vi "Word cmd.vi"(6 "Word cmd":T3, 8 "Error In (no error)":errorcluster, 10 "Mathcad Output":T1, 11 "DesignRequest":T2) -> (0 "error out":errorcluster, 1 "Find-Replace":cluster{"Find":string, "Replace":string}[](array[cluster]))   [LabVIEW 2012, in "Design Server.lvlib"]
uses:
  Design Server.lvlib
  Word cmd.ctl
  Design Request.ctl
  Variable cluster.ctl
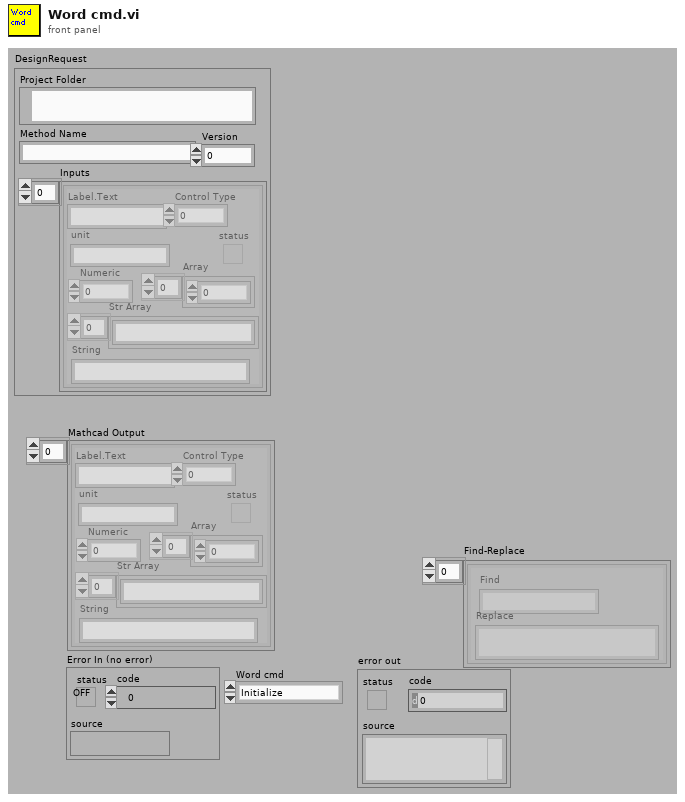
[diagram p1: front panel]
types:
  T1 = typedef "Design Server.lvlib/Variable cluster.ctl" = cluster{"Label.Text":string, "Control Type":u32, "Numeric":dbl, "Array":dbl[], "status":bool, "Str Array":string[], "String":string, "unit":string}[]
  T2 = typedef "Design Server.lvlib/Design Request.ctl" = cluster{"Project Folder":path, "Method Name":string, "Inputs":T1, "Version":i32}
  T3 = typedef "Design Server.lvlib/Word cmd.ctl" = enum16{"Initialize", "Create Reports", "Quit"}
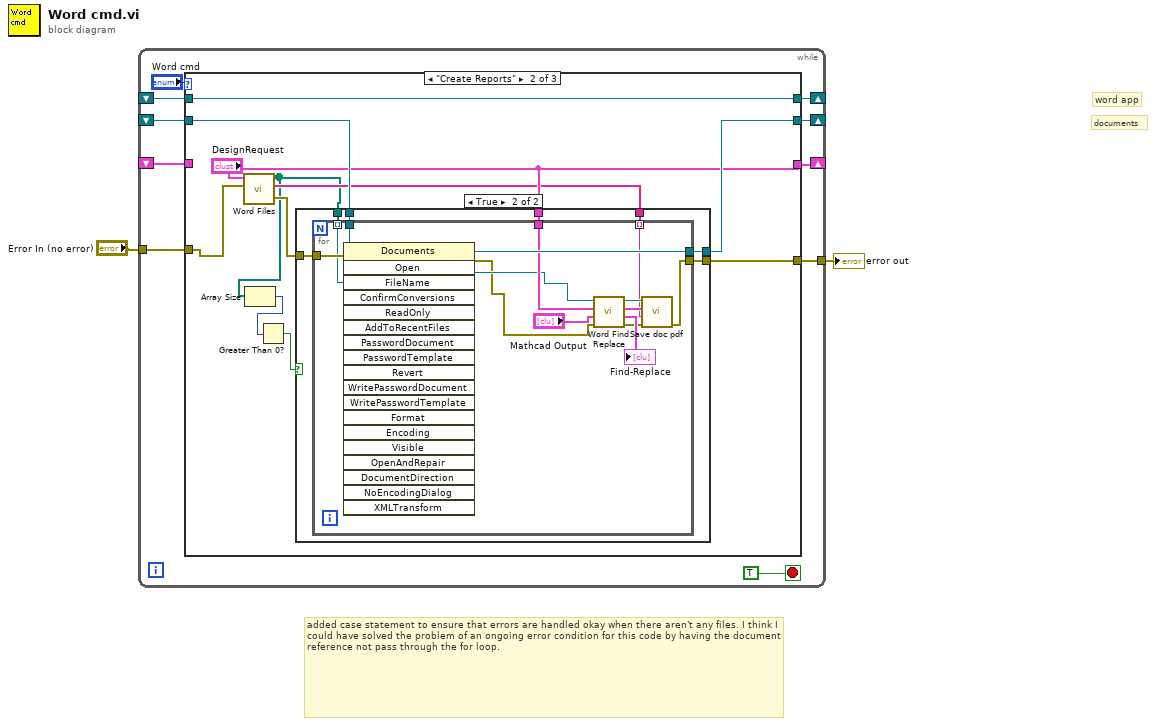
[diagram p0: block diagram]
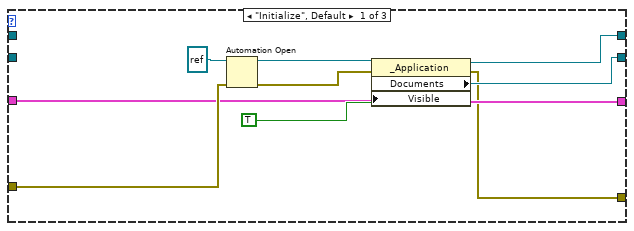
[diagram p2: hidden frame]
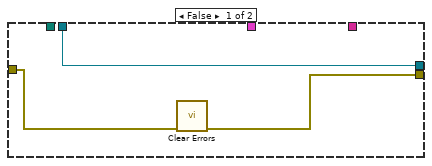
[diagram p3: hidden frame]
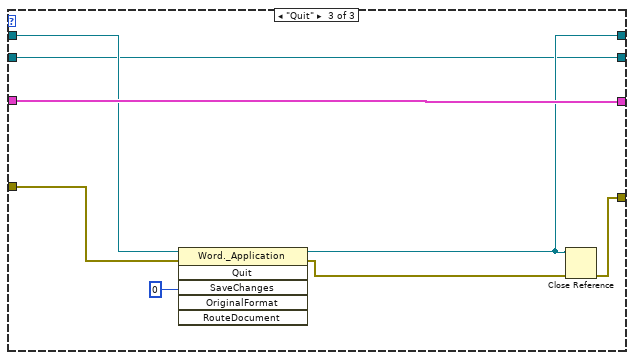
[diagram p4: hidden frame]
diagram:
  # "added case statement to ensure that errors are handled okay when there aren't any files. I think I could have solved the problem of an ongoing error condition for this code by having the document reference not pass through the for loop."
  # "documents"
  # "word app"
  n1 = while {
    shift-right: [w10] -> _
    shift-left: _ -> [w7]
    shift-right: [w9] -> _
    shift-left: _ -> [w8]
    tunnel: "Error In (no error)" -> [w6]
    tunnel: [w5] -> w1
    shift-right: [w4] -> _
    shift-left: _ -> [w3]
    stop <- TRUE stop-if-true
    n2 = case shown="\"Create Reports\"" "Word cmd" {
      tunnel: [w17 w27 w61] -> w10
      tunnel: [w16 w31 w58] -> w9
      tunnel: w8 -> [_ w32 w58]
      tunnel: w7 -> [_ w27 w63]
      tunnel: w6 -> [w15 w26 w60]
      tunnel: [w13 w30 w57] -> w5
      tunnel: [w14 "DesignRequest" w64] -> w4
      tunnel: w3 -> [w14 _ w64]
      frame "Initialize", Default {
        n3 = Automation Open(error in (no error)=w15, Automation Refnum=refnum<k7> refnum ("Word._Application")) -> (Automation Refnum=w21:refnum<k7>, error out=w20:errorcluster)  [unwired: 2 in]
        n4 = property class="_Application"(reference=w21, error in=w20, "Visible"=TRUE) -> (reference out=w17:refnum<k7>, error out=w13:errorcluster, "Documents"=w16:refnum<k7>)
      }
      frame "Create Reports" {
        n5 = call "Word Files.vi"("error in"=w26, "DesignRequest"="DesignRequest") -> ("filenames"=w28:string[], "Word Files"=w22:path[], "error out"=w25:errorcluster)  [unwired: 7 in]
        n6 = Array Size(array=w22) -> (size(s)=w24:i32)
        n7 = Greater Than 0?(x=w24) -> (x > 0?=w23:bool)
        n8 = case shown="True" w23 {
          tunnel: w32 -> [w34 w42]
          tunnel: [w34 w41] -> w31
          tunnel: [w33 w40] -> w30
          tunnel: "DesignRequest" -> [_ w39]
          tunnel: w22 -> [_ w38]
          tunnel: w28 -> [_ w37]
          tunnel: w25 -> [w35 w36]
          frame False {
            n9 = call <vilib>:"Clear Errors.vi"("error in (no error)"=w35) -> ("error out"=w33:errorcluster)  [unwired: 6 in]
          }
          frame True {
            n10 = for {
              tunnel: w42 -> [w56]
              tunnel: [w55] -> w41
              tunnel: [w44] -> w40
              tunnel: w36 -> [w54]
              tunnel: w38 -> [w53] mode=indexing
              tunnel: w39 -> [w52]
              tunnel: w37 -> [w43] mode=indexing
              n11 = invoke class="Documents" method="Open"(reference=w56, error in=w54, "FileName"=w53) -> (reference out=w55:refnum<k7>, error out=w45:errorcluster, "Open"=w50:refnum<k7>)  [unwired: 16 in, 16 out]
              n12 = call "Word Find Replace.vi"("error in (no error)"=w45, "Mathcad Output"="Mathcad Output", "DesignRequest"=w52, "Word Doc"=w50) -> ("error out"=w48:errorcluster, "Find-Replace"=→"Find-Replace":cluster{"Find":string, "Replace":string}[], "DesignRequest out"=w47:T2, "Word Doc out"=w46:refnum<k7>)  [unwired: 4 in]
              n13 = call "Save doc pdf.vi"("error in (no error)"=w48, "File Name"=w43, "DesignRequest"=w47, "ActiveDocument"=w46) -> ("error out"=w44:errorcluster)  [unwired: 7 in]
            }
          }
        }
      }
      frame "Quit" {
        n14 = invoke class="Word._Application" method="Quit"(reference=w63, error in=w60, "SaveChanges"=0) -> (reference out=w61:refnum<k7>, error out=w59:errorcluster)  [unwired: 3 in, 4 out]
        n15 = Close Reference(reference=w61, error in (no error)=w59) -> (error out=w57:errorcluster)
      }
    }
  }
  "error out" <- w1
